vi "Position AE.vi"(3 "Locked Position in":cluster{"X":dbl, "Y":dbl, "dx - dy":dbl}, 4 "Current Position in":cluster{"X":dbl, "Y":dbl, "dx - dy":dbl}, 5 "Action":T1) -> (0 "Locked Position out":cluster{"X":dbl, "Y":dbl, "dx - dy":dbl}, 1 "Current Position out":cluster{"X":dbl, "Y":dbl, "dx - dy":dbl})   [LabVIEW 2014]
uses:
  Controls/Standard Action for Position.ctl
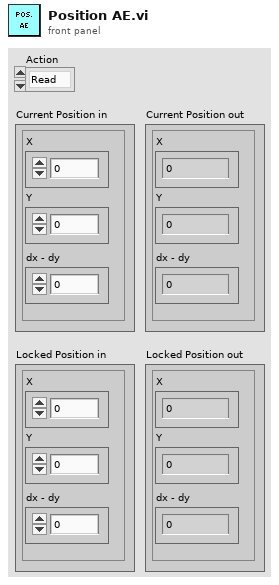
[diagram p1: front panel]
types:
  T1 = typedef "Standard Action for Position.ctl" = enum16{"Read", "Write Current", "Write Lock"}
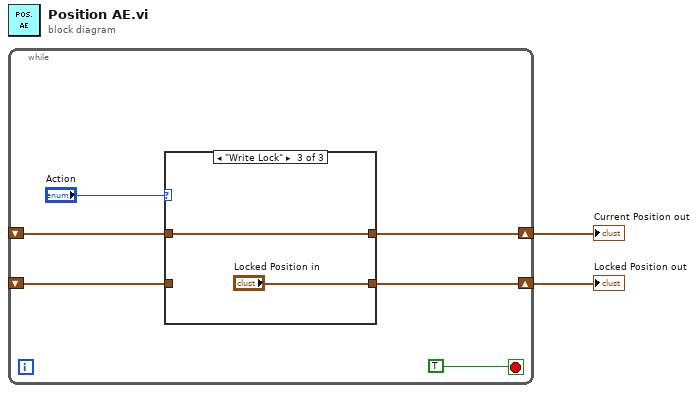
[diagram p0: block diagram]
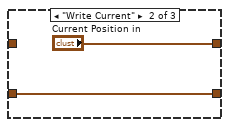
[diagram p3: hidden frame]
diagram:
  n1 = while {
    shift-right: [w8] -> w2
    shift-left: _ -> [w7]
    shift-right: [w5] -> w1
    shift-left: _ -> [w4]
    stop <- TRUE stop-if-true
    n2 = case shown="\"Write Lock\"" "Action" {
      tunnel: [w10 "Current Position in" w14] -> w8
      tunnel: w7 -> [w10 _ w14]
      tunnel: [w9 w11 "Locked Position in"] -> w5
      tunnel: w4 -> [w9 w11 _]
      frame "Read", Default {
      }
      frame "Write Current" {
      }
      frame "Write Lock" {
      }
    }
  }
  "Current Position out" <- w2
  "Locked Position out" <- w1
